vi "GDSIconEditor_ShrinkImage.vi"(10 "image data":T1) -> (3 "image subset":T1)   [LabVIEW 2020]
uses:
  <vilib>/picture/picture.llb/imagedata.ctl
panel:
  out "2D Picture 2":picture
  out "2D Picture":picture
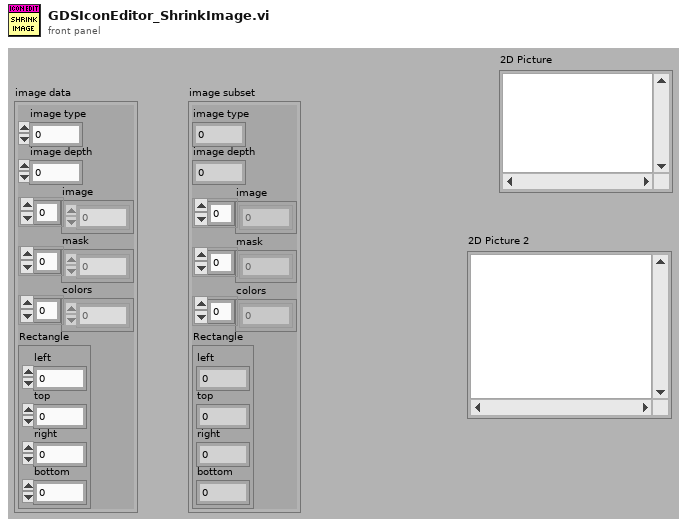
[diagram p1: front panel]
types:
  T1 = typedef "imagedata.ctl" = cluster{"image type":i32, "image depth":i32, "image":u8[], "mask":u8[], "colors":u32[], "Rectangle":cluster{"left":i16, "top":i16, "right":i16, "bottom":i16}}
  T2 = cluster{"left":i16, "top":i16, "right":i16, "bottom":i16}
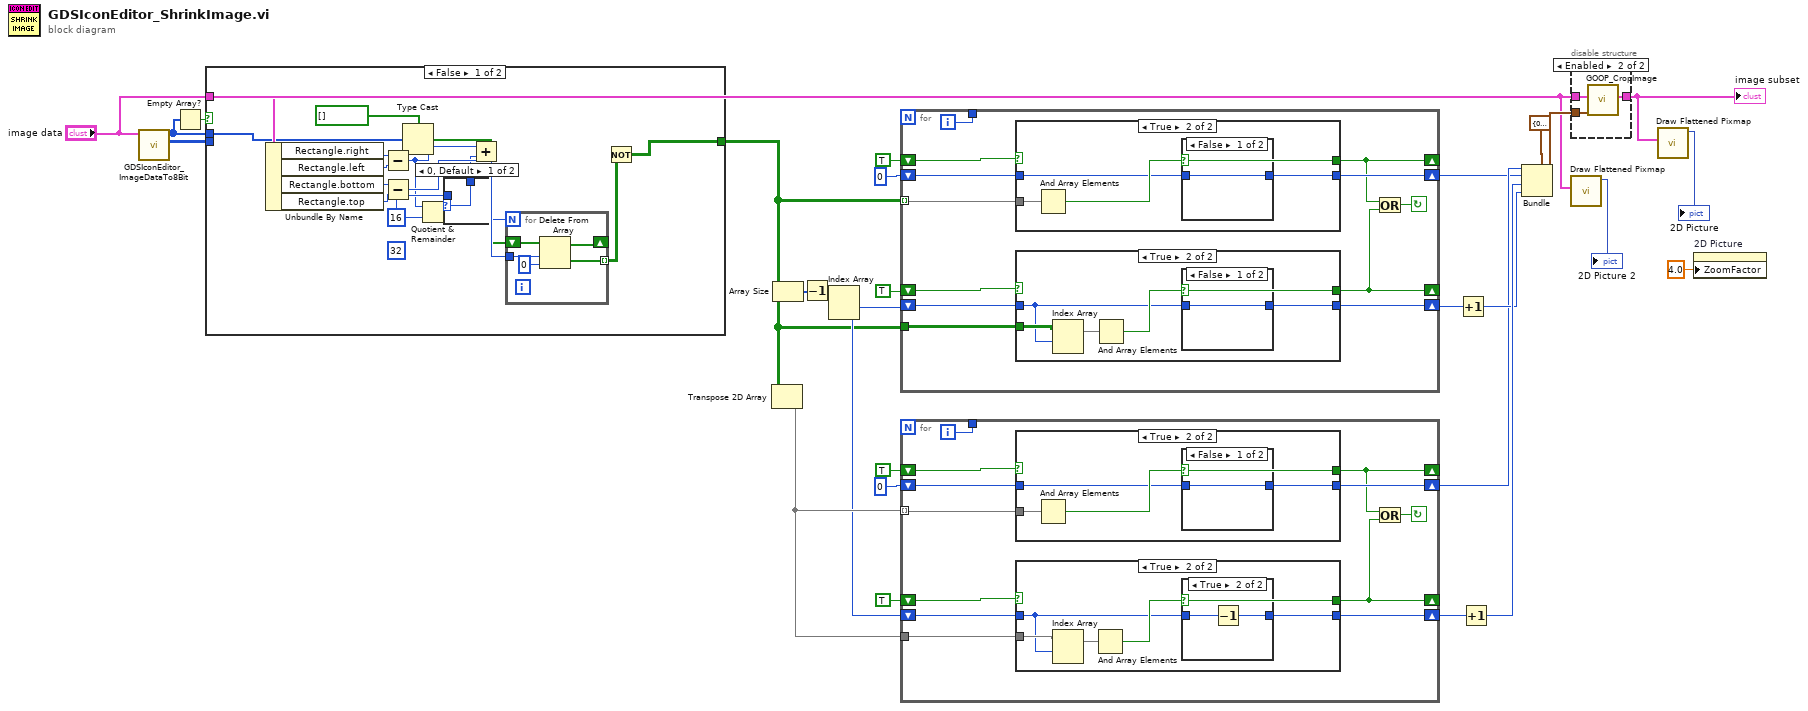
[diagram p0: block diagram]
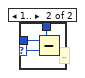
[diagram p2: hidden frame]
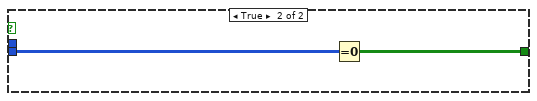
[diagram p3: hidden frame]
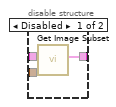
[diagram p4: hidden frame]
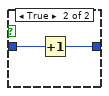
[diagram p8: hidden frame]
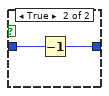
[diagram p10: hidden frame]
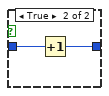
[diagram p12: hidden frame]
diagram:
  n1 = call "GDSIconEditor_ImageDataTo8Bit.vi"("image data"="image data") -> ("8-bit pixmap"=w8:u8[][], "mask"=w1:u8[])  [unwired: 7 in, 2 out]
  n2 = Empty Array?(array=w1) -> (empty?=w3:bool)
  n3 = case shown="False" w3 {
    tunnel: [w30 w55] -> w9
    tunnel: w8 -> [_ w54]
    tunnel: "image data" -> [w32 _]
    tunnel: w1 -> [w31 _]
    frame False {
      (unwired) i16 32 ("y")
      w41 = i16 16 ("y")
      n4 = Unbundle By Name(w32) -> ("Rectangle.right"=w34:i16, "Rectangle.left"=w35:i16, "Rectangle.bottom"=w36:i16, "Rectangle.top"=w37:i16)
      n5 = Subtract(x=w34, y=w35) -> (x-y=w38:i16)
      n6 = Subtract(x=w36, y=w37) -> (x-y=w42:i16)
      n7 = Type Cast(type=bool[] [], x=w31) -> (*(type *) &x=w43:bool[])
      n8 = Quotient & Remainder(x=w38, y=w41) -> (x-y*floor(x/y)=w39:i16)  [unwired: 1 out]
      n9 = case shown="0, Default" w39 {
        selector: w39 -> [w45 w48]
        tunnel: [w45 w47] -> w40
        tunnel: w41 -> [_ w46]
        frame 0, Default {
        }
        frame 1.. {
          # ".."
          n10 = Subtract(x=w46, y=w48) -> (x-y=w47:i16)
        }
      }
      n11 = Add(x=w38, y=w40) -> (x+y=w44:i16)
      n12 = for {
        N: w42 -> [_]
        shift-right: [w52] -> _
        shift-left: w43 -> [w53]
        tunnel: w44 -> [w50]
        tunnel: [w49] -> w29 mode=indexing
        n13 = Delete From Array(array=w53, length=w50, index=0) -> (deleted portion=w49:bool[], array with subset deleted=w52:bool[])
      }
      n14 = Not(x=w29) -> (.not. x?=w30:bool[][])
    }
    frame True {
      n15 = Equal To 0?(x=w54) -> (x = 0?=w55:bool[][])
    }
  }
  n16 = Transpose 2D Array(2D array=w9) -> (transposed array=w25:bool[][])
  n17 = Array Size(array=w9) -> (size(s)=w19:i32[])
  n18 = Decrement(x=w19) -> (x-1=w20:i32[])
  n19 = Index Array(array=w20) -> (element #1=w21:i32, element #2=w22:i32)  [unwired: 2 in]
  n20 = for {
    tunnel: w9 -> [w67] mode=indexing
    tunnel: w9 -> [w57]
    shift-right: [w64] -> w14
    shift-left: 0 -> [w65]
    shift-right: [w63] -> _
    shift-left: TRUE -> [w66]
    shift-right: [w61] -> w15
    shift-left: w21 -> [w60]
    shift-right: [w58] -> _
    shift-left: TRUE -> [w59]
    tunnel: [w56] -> _
    i -> [w56]
    stop <- w62 continue-if-true
    n21 = case shown="True" w66 {
      selector: w66 -> [w78 _]
      tunnel: w67 -> [_ w83]
      tunnel: w65 -> [w79 w81]
      tunnel: [w79 w80] -> w64
      tunnel: [w78 w82] -> w63
      frame False {
      }
      frame True {
        n22 = And Array Elements(Boolean array=w83) -> (logical AND=w82:bool)
        n23 = case shown="False" w82 {
          tunnel: w81 -> [w84 w86]
          tunnel: [w84 w85] -> w80
          frame False {
          }
          frame True {
            n24 = Increment(x=w86) -> (x+1=w85:i32)
          }
        }
      }
    }
    n25 = case shown="True" w59 {
      selector: w59 -> [w68 _]
      tunnel: w60 -> [w69 w71]
      tunnel: [w69 w73] -> w61
      tunnel: [w68 w74] -> w58
      tunnel: w57 -> [_ w72]
      frame False {
      }
      frame True {
        n26 = Index Array(array=w72, index (row)=w71) -> (element=w70:bool[])  [unwired: 1 in]
        n27 = And Array Elements(Boolean array=w70) -> (logical AND=w74:bool)
        n28 = case shown="False" w74 {
          tunnel: w71 -> [w75 w77]
          tunnel: [w75 w76] -> w73
          frame False {
          }
          frame True {
            n29 = Decrement(x=w77) -> (x-1=w76:i32)
          }
        }
      }
    }
    n30 = Or(x=w63, y=w58) -> (x .or. y?=w62:bool)
  }
  n31 = for {
    tunnel: w25 -> [w98] mode=indexing
    tunnel: w25 -> [w88]
    shift-right: [w95] -> w23
    shift-left: 0 -> [w96]
    shift-right: [w94] -> _
    shift-left: TRUE -> [w97]
    shift-right: [w92] -> w24
    shift-left: w22 -> [w91]
    shift-right: [w89] -> _
    shift-left: TRUE -> [w90]
    tunnel: [w87] -> _
    i -> [w87]
    stop <- w93 continue-if-true
    n32 = case shown="True" w97 {
      selector: w97 -> [w109 _]
      tunnel: w98 -> [_ w114]
      tunnel: w96 -> [w110 w112]
      tunnel: [w110 w111] -> w95
      tunnel: [w109 w113] -> w94
      frame False {
      }
      frame True {
        n33 = And Array Elements(Boolean array=w114) -> (logical AND=w113:bool)
        n34 = case shown="False" w113 {
          tunnel: w112 -> [w115 w117]
          tunnel: [w115 w116] -> w111
          frame False {
          }
          frame True {
            n35 = Increment(x=w117) -> (x+1=w116:i32)
          }
        }
      }
    }
    n36 = case shown="True" w90 {
      selector: w90 -> [w99 _]
      tunnel: w91 -> [w100 w102]
      tunnel: [w100 w104] -> w92
      tunnel: [w99 w105] -> w89
      tunnel: w88 -> [_ w103]
      frame False {
      }
      frame True {
        n37 = Index Array(array=w103, index (row)=w102) -> (element=w101:bool[])  [unwired: 1 in]
        n38 = And Array Elements(Boolean array=w101) -> (logical AND=w105:bool)
        n39 = case shown="True" w105 {
          tunnel: w102 -> [w106 w108]
          tunnel: [w106 w107] -> w104
          frame False {
          }
          frame True {
            n40 = Decrement(x=w108) -> (x-1=w107:i32)
          }
        }
      }
    }
    n41 = Or(x=w94, y=w89) -> (x .or. y?=w93:bool)
  }
  n42 = Increment(x=w15) -> (x+1=w27:i32)
  n43 = Increment(x=w24) -> (x+1=w28:i32)
  n44 = Bundle(cluster=T2 {"left"=0, "top"=0, "right"=0, "bottom"=0} ("subset rect"), "left"=w23, "top"=w14, "right"=w28, "bottom"=w27) -> (w26:T2)
  n45 = call <vilib>:"Draw Flattened Pixmap.vi"("image data"="image data") -> ("new picture"=→"2D Picture 2":picture)  [unwired: 8 in]
  n46 = disable-structure shown="Enabled" {
    disable-tunnel: w26 -> [w120 w122]
    disable-tunnel: [w119 w121] -> w6
    disable-tunnel: "image data" -> [w118 w123]
    frame Disabled {
      n47 = call <vilib>:"Get Image Subset.vi"("subset rect"=w120, "image data"=w118) -> ("image subset"=w119:T1)  [unwired: 4 in, 1 out]
    }
    frame Enabled {
      n48 = call "GOOP_CropImage.vi"("subset rect"=w122, "image data"=w123) -> ("image subset"=w121:T1)  [unwired: 4 in, 1 out]
    }
  }
  "image subset" <- w6
  n49 = call <vilib>:"Draw Flattened Pixmap.vi"("image data"=w6) -> ("new picture"=→"2D Picture":picture)  [unwired: 8 in]
  n50 = property on="2D Picture" class="Pict"("ZoomFactor"=sgl 4.0 ("Zoom Factor")) -> ()  [unwired: 2 in, 2 out]
